vi "MAPP_Version.vi"(8 "error in (no error)":errorcluster) -> (0 "error out":errorcluster, 1 "FileVersionInfo Out":T1, 2 "Application Path out":path, 3 "File Version Info":string)   [LabVIEW 2018]
uses:
  <vilib>/Platform/fileVersionInfo.llb/FileVersionInformation.ctl
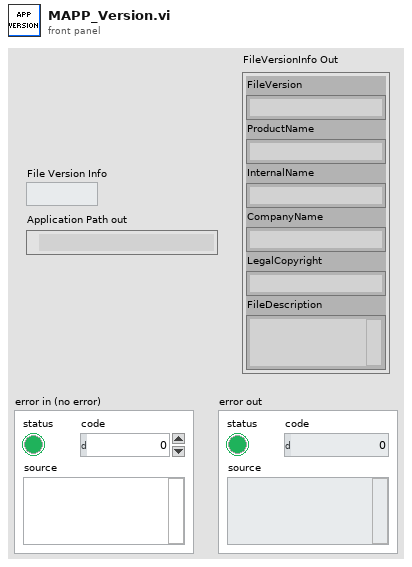
[diagram p1: front panel]
types:
  T1 = typedef "FileVersionInformation.ctl" = cluster{"FileVersion":string, "ProductName":string, "InternalName":string, "CompanyName":string, "LegalCopyright":string, "FileDescription":string}
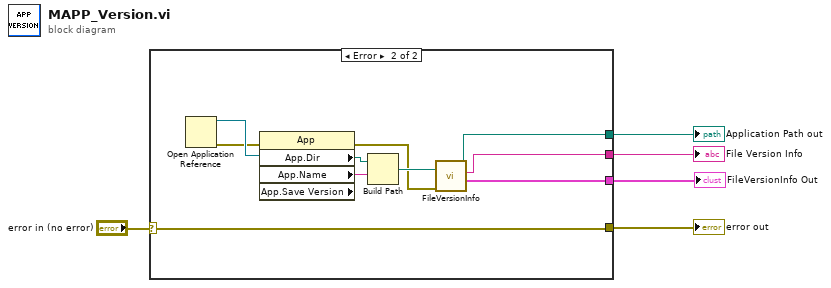
[diagram p0: block diagram]
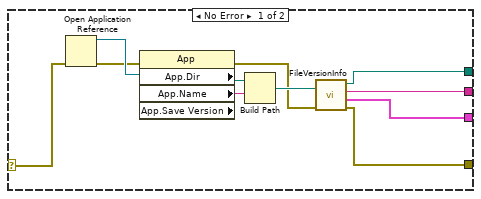
[diagram p2: hidden frame]
diagram:
  n1 = case shown="Error" "error in (no error)" {
    selector: "error in (no error)" -> [w8 w18]
    tunnel: [w16 w20] -> w5
    tunnel: [w15 w18] -> w4
    tunnel: [w7 w19] -> w2
    tunnel: [w6 w17] -> w1
    frame No Error {
      n2 = Open Application Reference(8:w8) -> (0:w11:errorcluster, 3:w14:refnum<vi>)  [unwired: 3 in]
      n3 = property class="App" props=["App.Dir", "App.Name", "App.Save Version"](reference=w14, error in=w11) -> (error out=w9:errorcluster, "App.Dir"=w13:path, "App.Name"=w12:string)  [unwired: 2 out]
      n4 = Build Path(base path=w13, name or relative path=w12) -> (appended path=w10:path)
      n5 = call <vilib>:"FileVersionInfo.vi"("error in (no error)"=w9, "Application Path in"=w10) -> ("error out"=w15:errorcluster, "FileVersionInfo Out"=w7:T1, "File Version Info"=w16:string, "Application Path out"=w6:path)  [unwired: 6 in]
    }
    frame Error {
      n6 = Open Application Reference() -> (0:w23:errorcluster, 3:w26:refnum<vi>)  [unwired: 4 in]
      n7 = property class="App" props=["App.Dir", "App.Name", "App.Save Version"](reference=w26, error in=w23) -> (error out=w21:errorcluster, "App.Dir"=w25:path, "App.Name"=w24:string)  [unwired: 2 out]
      n8 = Build Path(base path=w25, name or relative path=w24) -> (appended path=w22:path)
      n9 = call <vilib>:"FileVersionInfo.vi"("error in (no error)"=w21, "Application Path in"=w22) -> ("FileVersionInfo Out"=w19:T1, "File Version Info"=w20:string, "Application Path out"=w17:path)  [unwired: 6 in, 1 out]
    }
  }
  "File Version Info" <- w5
  "error out" <- w4
  "FileVersionInfo Out" <- w2
  "Application Path out" <- w1
